vi "draw_lanes_coord.vi"(4 "error in":errorcluster, 7 "monoDrive in":T1={"Config"={"Trajectory"={"Number of frames"=0, "Frame number"=0, "Trajectory"=""}, "Weather"={"id"=""}}, "Connections"={"Simulator Connection"=refnum, "server_ip"="127.0.0.1", "Port"=0, "Sensor connections"=[]}, "Map"={"lanes"={"x"=[], "y"=[], "z"=[]}, "StartPosition"={"start_points"={"locations"=[], "rotations"=[], "type"=[]}, "StartRotation"=[], "StartLocation"=[]}, "Draw Map Size"={"Width"=0, "Height"=0}, "DrawArea"={"min_Y"=0.0, "min_X"=0.0, "Scale X"=0.0, "Scale Y"=0.0}, "Map"=bytes[0], "Map Geojson"=""}}) -> (0 "error out":errorcluster, 3 "monoDrive out":T1={"Config"={"Trajectory"={"Number of frames"=0, "Frame number"=0, "Trajectory"=""}, "Weather"={"id"=""}}, "Connections"={"Simulator Connection"=refnum, "server_ip"="127.0.0.1", "Port"=0, "Sensor connections"=[]}, "Map"={"lanes"={"x"=[], "y"=[], "z"=[]}, "StartPosition"={"start_points"={"locations"=[], "rotations"=[], "type"=[]}, "StartRotation"=[], "StartLocation"=[]}, "Draw Map Size"={"Width"=0, "Height"=0}, "DrawArea"={"min_Y"=0.0, "min_X"=0.0, "Scale X"=0.0, "Scale Y"=0.0}, "Map"=bytes[0], "Map Geojson"=""}})   [LabVIEW 2019]
uses:
  controls/simx_connection.ctl
  controls/config.ctl
  controls/trajectory.ctl
  controls/weather.ctl
  controls/connections.ctl
  controls/start_points.ctl
  <vilib>/Utility/miscctls.llb/LVBoundsTypeDef.ctl
panel:
  out "map":picture
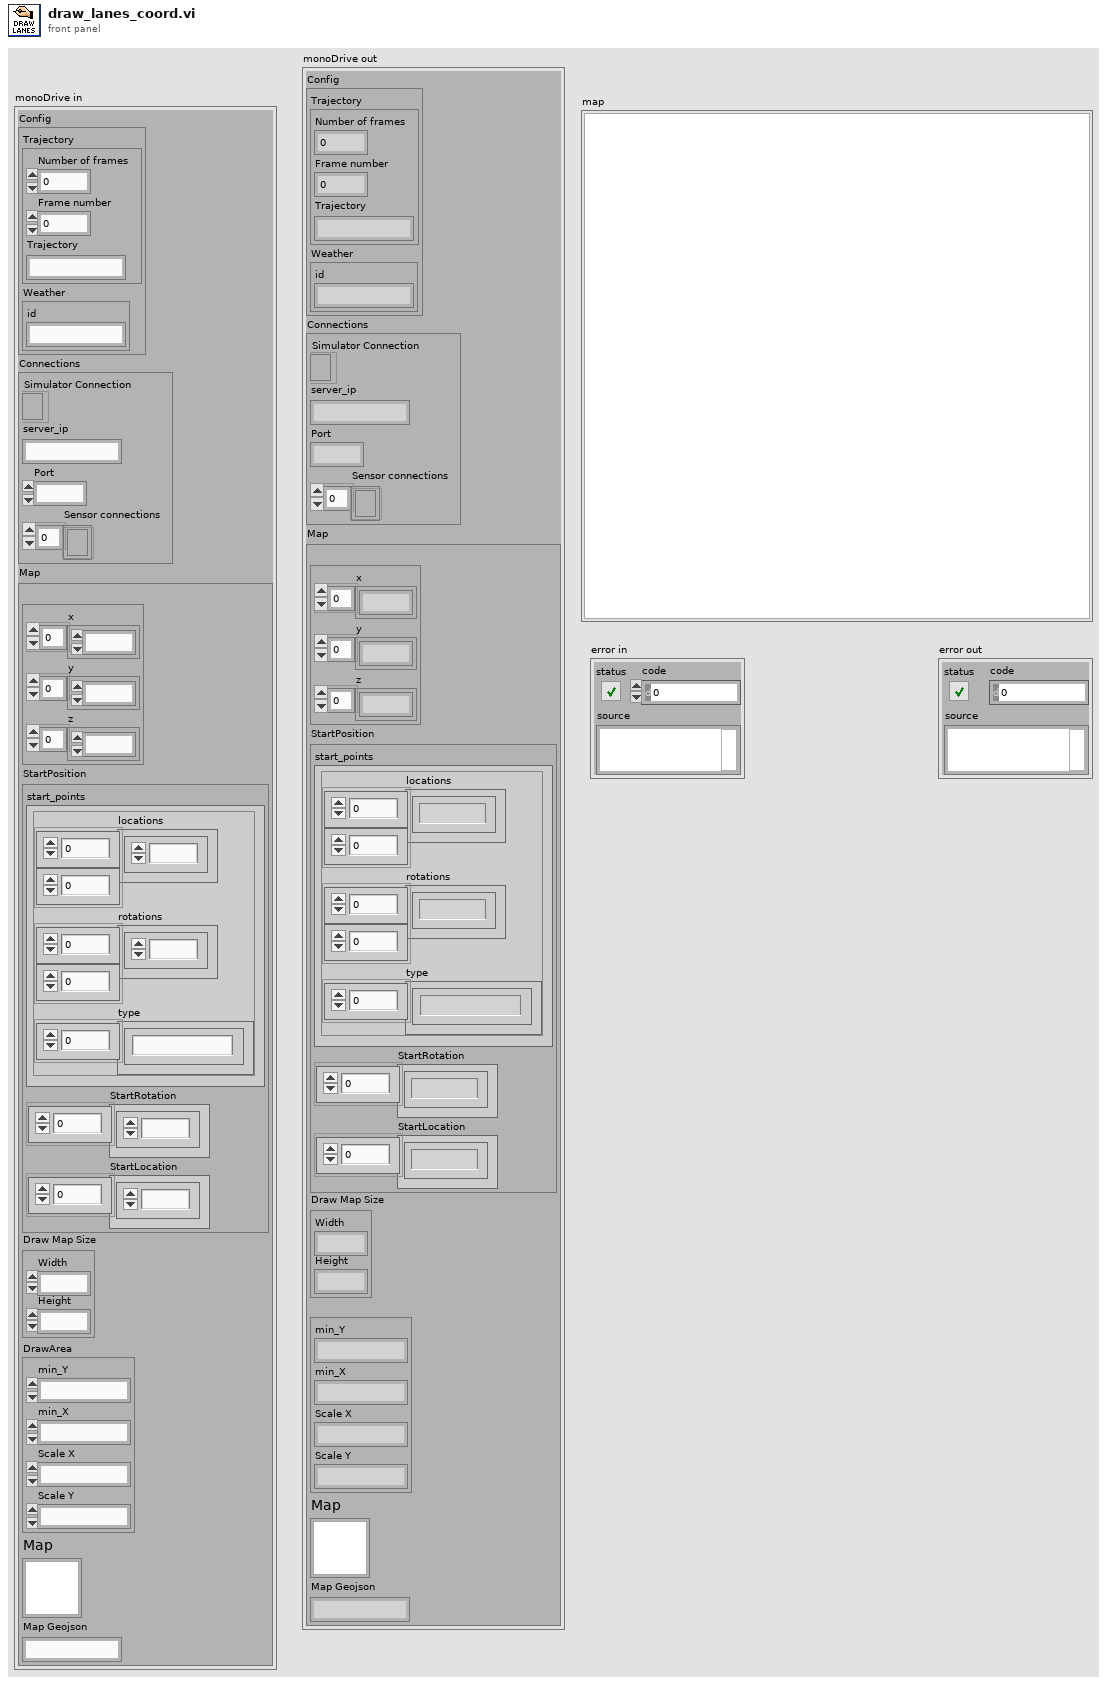
[diagram p1: front panel]
types:
  T1 = typedef "simx_connection.ctl" = cluster{"Config":T2, "Connections":T5, "Map":cluster{"lanes":cluster{"x":dbl[], "y":dbl[], "z":dbl[]}, "StartPosition":cluster{"start_points":T6, "StartRotation":dbl[], "StartLocation":dbl[]}, "Draw Map Size":T7, "DrawArea":cluster{"min_Y":dbl, "min_X":dbl, "Scale X":dbl, "Scale Y":dbl}, "Map":picture, "Map Geojson":string}}
  T2 = typedef "config.ctl" = cluster{"Trajectory":T3, "Weather":T4}
  T3 = typedef "trajectory.ctl" = cluster{"Number of frames":i32, "Frame number":i32, "Trajectory":string}
  T4 = typedef "weather.ctl" = cluster{"id":string}
  T5 = typedef "connections.ctl" = cluster{"Simulator Connection":refnum<k5>, "server_ip":string, "Port":i32, "Sensor connections":refnum<k5>[]}
  T6 = typedef "start_points.ctl" = cluster{"locations":dbl[][], "rotations":dbl[][], "type":string[]}
  T7 = typedef "LVBoundsTypeDef.ctl" = cluster{"Width":u32, "Height":u32}
  T8 = cluster{"min_Y":dbl, "min_X":dbl, "Scale X":dbl, "Scale Y":dbl}
  T9 = cluster{"Width":u16, "Style":enum32{"Solid", "Dash", "Dot", "DashDot", "DashDotDot"}}
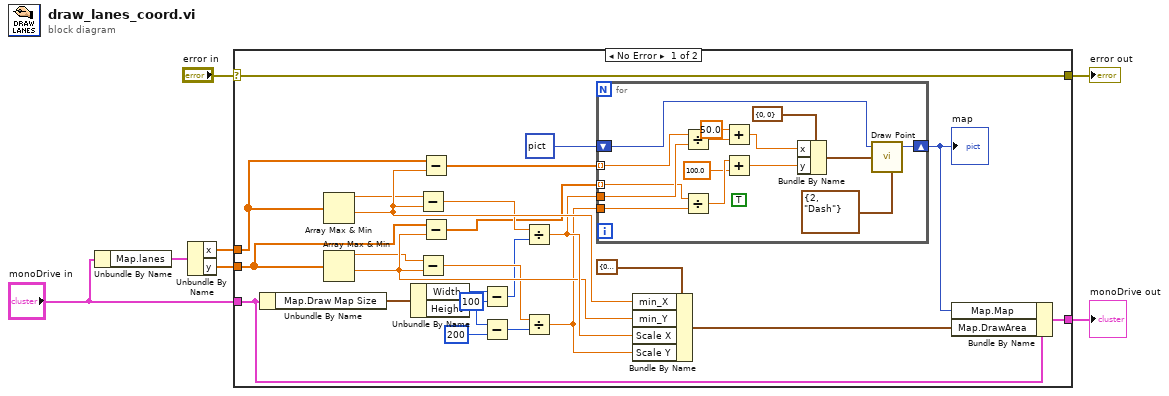
[diagram p0: block diagram]
diagram:
  n1 = Unbundle By Name("monoDrive in") -> ("Map.lanes"=w7:cluster{"x":dbl[], "y":dbl[], "z":dbl[]})
  n2 = Unbundle By Name(w7) -> ("x"=w6:dbl[], "y"=w1:dbl[])
  n3 = case shown="No Error" "error in" {
    selector: "error in" -> [w32 w50]
    tunnel: [w32 w50] -> w3
    tunnel: w1 -> [w20 _]
    tunnel: w6 -> [w22 _]
    tunnel: "monoDrive in" -> [w24 w49]
    tunnel: [w26 w49] -> w5
    frame No Error {
      n4 = Unbundle By Name(w24) -> ("Map.Draw Map Size"=w23:T7)
      n5 = Array Max & Min(array=w22) -> (max value=w19:dbl, min value=w31:dbl)  [unwired: 2 out]
      n6 = Array Max & Min(array=w20) -> (max value=w15:dbl, min value=w18:dbl)  [unwired: 2 out]
      n7 = Unbundle By Name(w23) -> ("Width"=w11:u32, "Height"=w10:u32)
      n8 = Subtract(x=w19, y=w31) -> (x-y=w30:dbl)
      n9 = Subtract(x=w15, y=w18) -> (x-y=w17:dbl)
      n10 = Subtract(x=w22, y=w31) -> (x-y=w21:dbl[])
      n11 = Subtract(x=w20, y=w18) -> (x-y=w16:dbl[])
      n12 = Subtract(x=w11, y=u32 100) -> (x-y=w13:u32)
      n13 = Subtract(x=w10, y=u32 200 ("x")) -> (x-y=w12:u32)
      n14 = Divide(x=w30, y=w13) -> (x/y=w29:dbl)
      n15 = Divide(x=w17, y=w12) -> (x/y=w14:dbl)
      n16 = for {
        shift-right: [w48] -> w25
        shift-left: picture data[5B] ("new picture") -> [w47]
        tunnel: w29 -> [w43]
        tunnel: w21 -> [w42] mode=indexing
        tunnel: w16 -> [w41] mode=indexing
        tunnel: w14 -> [w38]
        (unwired) TRUE ("absolute coordinates?(T)")
        n17 = Divide(x=w42, y=w43) -> (x/y=w40:dbl)
        n18 = Divide(x=w41, y=w38) -> (x/y=w39:dbl)
        n19 = Add(x=50.0, y=w40) -> (x+y=w36:dbl)
        n20 = Add(x=w39, y=100.0) -> (x+y=w37:dbl)
        n21 = Bundle By Name(cluster=cluster{"x":i16, "y":i16} {"x"=0, "y"=0} ("point(x,y)"), "x"=w36, "y"=w37) -> (w45:cluster{"x":i16, "y":i16})
        n22 = call <vilib>:"Draw Point.vi"("picture"=w47, "point(x,y)"=w45, "pen"=T9 {"Width"=2, "Style"=enum."Dash"}) -> ("new picture"=w48:picture)  [unwired: 6 in]
      }
      "map" <- w25
      n23 = Bundle By Name(cluster=T8 {"min_Y"=0.0, "min_X"=0.0, "Scale X"=0.0, "Scale Y"=0.0} ("Map.DrawArea"), "min_X"=w31, "min_Y"=w18, "Scale X"=w29, "Scale Y"=w14) -> (w27:T8)
      n24 = Bundle By Name(cluster=w24, "Map.Map"=w25, "Map.DrawArea"=w27) -> (w26:T1)
    }
    frame Error {
    }
  }
  "error out" <- w3
  "monoDrive out" <- w5
